vi "JoystickControls.vi"() -> (3 "input cluster":T1)   [LabVIEW 2015]
uses:
  Controls.ctl
  References/Refnums.vi
  <vilib>/Rock Robotics/WPI/Utilities/WPI_GetSetVariantRefNum.vi
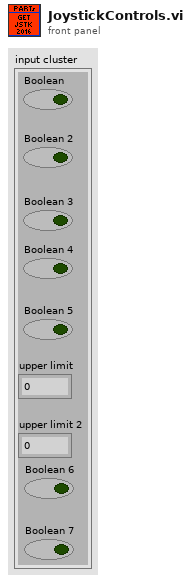
[diagram p1: front panel]
types:
  T1 = typedef "Controls.ctl" = cluster{"Boolean":bool, "Boolean 2":bool, "Boolean 3":bool, "Boolean 4":bool, "Boolean 5":bool, "upper limit":dbl, "upper limit 2":dbl, "Boolean 6":bool, "Boolean 7":bool}
  T2 = typedef "WPI_JoystickDevRef.ctl" = cluster{"Device":T3}
  T3 = typedef "WPI_JoystickDeviceEnum.ctl" = enum16{"USB 0", "USB 1", "USB 2", "USB 3", "USB 4", "USB 5"}
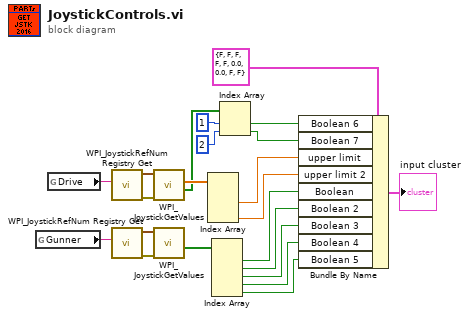
[diagram p0: block diagram]
diagram:
  n1 = global read "Refnums.vi" "Gunner"() -> (w21:string)
  n2 = global read "Refnums.vi" "Drive"() -> (w20:string)
  n3 = call <vilib>:"WPI_JoystickRefNum Registry Get.vi"("refnum name"=w20) -> ("error out"=w19:errorcluster, "JoystickDevRef"=w18:T2)  [unwired: 9 in]
  n4 = call <vilib>:"WPI_JoystickRefNum Registry Get.vi"("refnum name"=w21) -> ("error out"=w16:errorcluster, "JoystickDevRef"=w17:T2)  [unwired: 9 in]
  n5 = call <vilib>:"WPI_JoystickGetValues.vi"("error in (no error)"=w19, "JoystickDevRef"=w18) -> ("Buttons"=w7:bool[], "Axes"=w8:dbl[])  [unwired: 5 in, 3 out]
  n6 = call <vilib>:"WPI_JoystickGetValues.vi"("error in (no error)"=w16, "JoystickDevRef"=w17) -> ("Buttons"=w22:bool[])  [unwired: 5 in, 4 out]
  n7 = Index Array(array=w8) -> (element #2=w2:dbl, element #4=w1:dbl)  [unwired: 4 in, 2 out]
  n8 = Index Array(array=w22) -> (element #1=w15:bool, element #2=w14:bool, element #3=w13:bool, element #4=w12:bool, element #5=w11:bool)  [unwired: 5 in]
  n9 = Index Array(array=w7, index #1=1 ("index"), index #2=2 ("index")) -> (element #1=w4:bool, element #2=w3:bool)
  n10 = Bundle By Name(cluster=T1 {"Boolean"=FALSE, "Boolean 2"=FALSE, "Boolean 3"=FALSE, "Boolean 4"=FALSE, "Boolean 5"=FALSE, "upper limit"=0.0, "upper limit 2"=0.0, "Boolean 6"=FALSE, "Boolean 7"=FALSE} ("input cluster"), "Boolean 6"=w4, "Boolean 7"=w3, "upper limit"=w2, "upper limit 2"=w1, "Boolean"=w15, "Boolean 2"=w14, "Boolean 3"=w13, "Boolean 4"=w12, "Boolean 5"=w11) -> (→"input cluster":T1)
